vi "RotatingFieldCalculation_uvw.vi"(8 "Time Step (ms)":sgl=1.0, 9 "Flux density magnitude (T)":sgl, 10 "Previous Field Angle (rad)":sgl, 11 "Omega (rad/s)":sgl) -> (1 "Bv (T)":sgl, 2 "Bu (T)":sgl, 3 "New Field Angle (rad)":sgl)   [LabVIEW 2020]
panel:
  # "User inputs"
  # "Control parameters"
  # "Output"
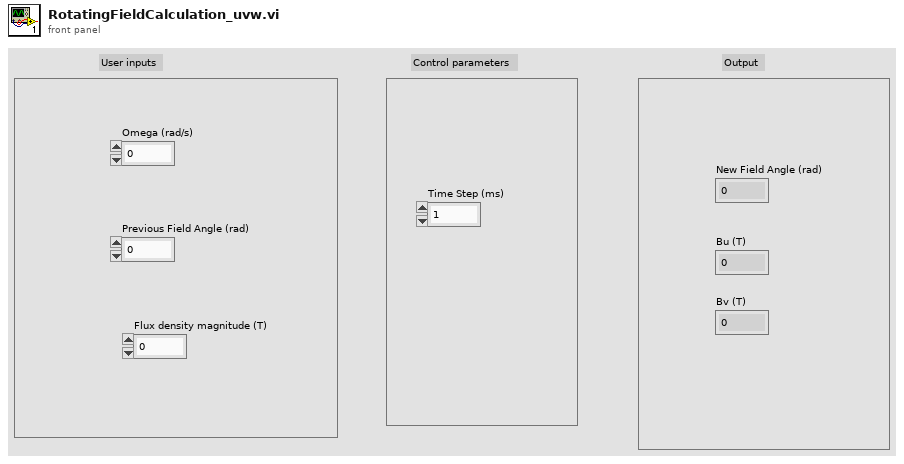
[diagram p1: front panel]
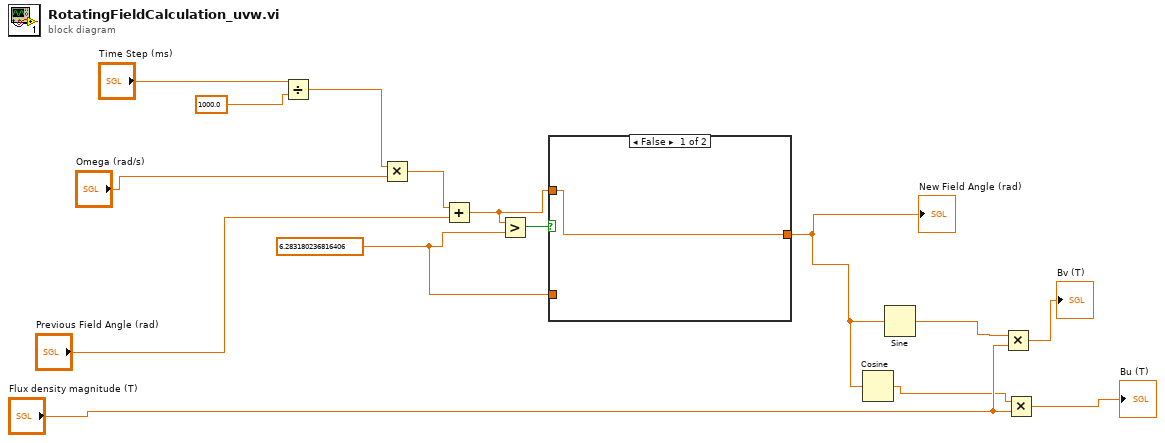
[diagram p0: block diagram]
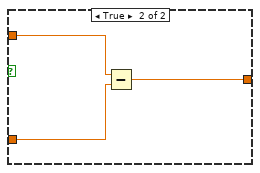
[diagram p2: hidden frame]
diagram:
  w7 = sgl 6.28318
  n1 = Divide(x="Time Step (ms)", y=sgl 1000.0) -> (x/y=w14:sgl)
  n2 = Multiply(x=w14, y="Omega (rad/s)") -> (x*y=w11:sgl)
  n3 = Add(x=w11, y="Previous Field Angle (rad)") -> (x+y=w8:sgl)
  n4 = Greater?(x=w8, y=w7) -> (0:w9:bool)
  n5 = case shown="False" w9 {
    tunnel: w8 -> [w16 w19]
    tunnel: w7 -> [_ w18]
    tunnel: [w16 w17] -> w1
    frame False {
    }
    frame True {
      n6 = Subtract(x=w19, y=w18) -> (x-y=w17:sgl)
    }
  }
  "New Field Angle (rad)" <- w1
  n7 = Cosine(x=w1) -> (cos(x)=w3:sgl)
  n8 = Sine(x=w1) -> (sin(x)=w2:sgl)
  n9 = Multiply(x=w2, y="Flux density magnitude (T)") -> (x*y=→"Bv (T)":sgl)
  n10 = Multiply(x=w3, y="Flux density magnitude (T)") -> (x*y=→"Bu (T)":sgl)
